vi "Test Find Two Missing Chars.vi"(11 "Test Case In":refnum<class "Removed Section Finder Test.lvclass">) -> (0 "error out":errorcluster, 3 "Test Case Out":refnum<class "Removed Section Finder Test.lvclass">)   [LabVIEW 2020, in "Removed Section Finder Test.lvclass"]
uses:
  Removed Section Finder Test.lvclass
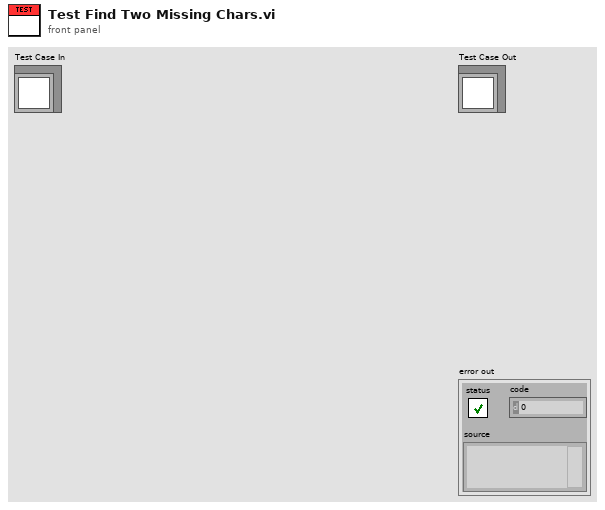
[diagram p1: front panel]
types:
  T1 = cluster{"Selection Start":u32, "Selection End":u32}
  T2 = cluster{"Selection Start":u32, "Selection End":u32}[]
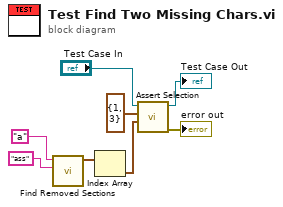
[diagram p0: block diagram]
diagram:
  n1 = call "Find Removed Sections.vi"("Reference"="ass", "Target"="a") -> ("Sections in Reference"=w2:T2)  [unwired: 9 in]
  n2 = Index Array(array=w2) -> (element=w1:T1)  [unwired: 1 in]
  n3 = call "Assert Selection.vi"("Actual"=w1, "Expected"=T1 {"Selection Start"=1, "Selection End"=3} ("Missmatches"), "Removed Section Finder Test In"="Test Case In") -> ("error out"=→"error out":errorcluster, "Removed Section Finder Test Out"=→"Test Case Out":refnum<class "Removed Section Finder Test.lvclass">)  [unwired: 7 in]
